vi "ExpandArray.vi"(10 "Scale Factor":u16, 11 "Input AO Array":i16[](array[numeric])) -> (3 "Output Array":i16[](array[numeric]))   [LabVIEW 2021]
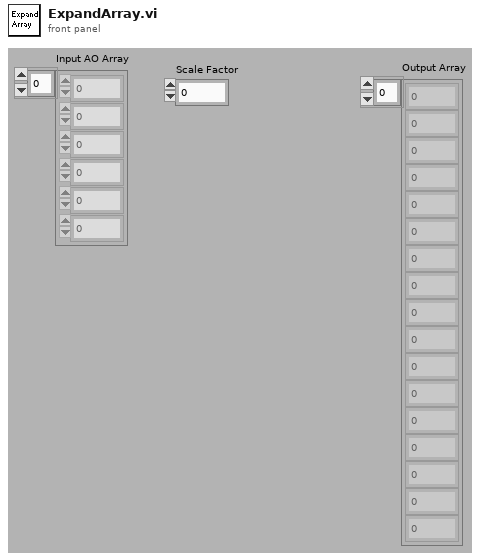
[diagram p1: front panel]
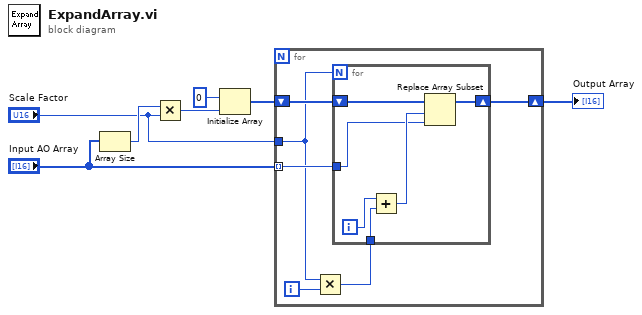
[diagram p0: block diagram]
diagram:
  n1 = Array Size(array="Input AO Array") -> (size(s)=w5:i32)
  n2 = Multiply(x=w5, y="Scale Factor") -> (x*y=w4:i32)
  n3 = Initialize Array(i16 0, w4) -> (w3:i16[])
  n4 = for {
    tunnel: "Input AO Array" -> [w12] mode=indexing
    shift-right: [w11] -> w1
    shift-left: w3 -> [w13]
    tunnel: "Scale Factor" -> [w9]
    i -> [w10]
    n5 = Multiply(x=w9, y=w10) -> (x*y=w8:i32)
    n6 = for {
      N: w9 -> [_]
      shift-right: [w18] -> w11
      shift-left: w13 -> [w19]
      tunnel: w12 -> [w15]
      tunnel: w8 -> [w14]
      i -> [w17]
      n7 = Add(x=w17, y=w14) -> (x+y=w16:i32)
      n8 = Replace Array Subset(array=w19, new element=w15, index=w16) -> (w18:i16[])
    }
  }
  "Output Array" <- w1
